vi "5017_18_Module_configure.vi"() -> ()   [LabVIEW 2010]
uses:
  ADAM Client/Sub VIs/ADAM Controls/Address.ctl
panel:
  out "Timed out":bool
  out "Serial Error":bool
  in  "Address (Main, Sub reqd.)":T1={"Main"=0, "Ch."=0, "Sub"=0, "Port Name"="MainNetwork"}
  in  "Range Setting":u16(ring)=15 items=["00     +/-15mV", "01     +/-50mV", "02     +/-100mV", "03     +/-500mV", "04     +/-1V", "05     +/-2.5V", "06     +/-20mA", "NOT USED", "08     +/-10V", "09     +/-5V", "0A     +/-1V", "0B     +/-500mV", "0C     +/-150mV", "0D     +/-20mA", "0E     Type J", "0F     Type K", "10     Type T", "11     Type E", "12     Type R", "13     Type S", "14     Type B"]
  in  "Data Format (ONLY ENG UNITS)":u16(ring) items=["Engineering Units", "% of FSR", "Hex", "Ohms (4013)"]
  in  "Mains Frquency":bool=TRUE
  out "Reply":string
  out "String to Write":string
  # "Happy reply starts \"!\"\nUnhappy reply starts \"?\""
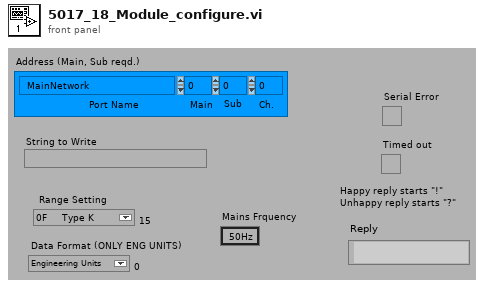
[diagram p1: front panel]
types:
  T1 = typedef "Address.ctl" = cluster{"Main":i32, "Ch.":i32, "Sub":i32, "Port Name":string}
  T2 = cluster{"Boolean array[0]":bool, "Boolean array[1]":bool}
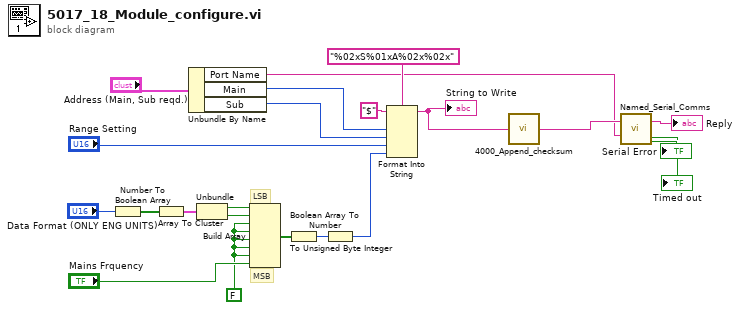
[diagram p0: block diagram]
diagram:
  w7 = FALSE
  # "MSB"
  # "LSB"
  n1 = Number To Boolean Array(number="Data Format (ONLY ENG UNITS)") -> (Boolean array=w14:bool[])
  n2 = Array To Cluster(array=w14) -> (cluster=w13:T2)
  n3 = Unbundle By Name("Address (Main, Sub reqd.)") -> ("Port Name"=w3:string, "Main"=w6:i32, "Sub"=w5:i32)
  n4 = Unbundle(w13) -> ("Boolean array[0]"=w12:bool, "Boolean array[1]"=w11:bool)
  n5 = Build Array(w12, w11, w7, w7, w7, w7, w7, "Mains Frquency") -> (w20:bool[])
  n6 = Boolean Array To Number(Boolean array=w20) -> (number=w19:u32)
  n7 = To Unsigned Byte Integer(number=w19) -> (unsigned 8bit integer=w4:u8)
  n8 = Format Into String(format string="%02xS%01xA%02x%02x", initial string="$", w6, w5, "Range Setting", w4) -> (resulting string=w18:string)  [unwired: 1 in, 1 out]
  "String to Write" <- w18
  n9 = call "4000_Append_checksum.vi"("ADAM command"=w18) -> ("ADAM string to send"=w9:string)
  n10 = call "Named_Serial_Comms.vi"("Write String"=w9, "Port Name"=w3) -> ("Read"=→"Reply":string, "Timed out"=→"Timed out":bool, "Serial Error"=→"Serial Error":bool)  [unwired: 10 in, 1 out]
